vi "Average.vi"(0 "Sonar name":string) -> (7 "Sum":dbl[](array[numeric]), 8 "Average":dbl)   [LabVIEW 2017]
uses:
  <vilib>/Rock Robotics/WPI/Ultrasonic/WPI_SonarMB1010AnalogRefNum Registry Get.vi
panel:
  # "Takes 10 numbers"
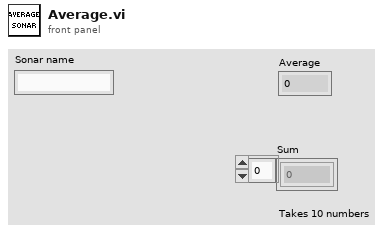
[diagram p1: front panel]
types:
  T1 = typedef "WPI_SonarMB1010AnalogDeviceRef.ctl" = cluster{"AIDeviceRef":T2, "Scaling factor (V/in)":dbl, "Average Bits":u8}
  T2 = typedef "WPI_AnalogChannelDevRef.ctl" = cluster{"DevStatus":errorcluster, "Analog Channel":T3}
  T3 = typedef "FPGA_AIChannel.ctl" = enum8{"AI 0", "AI 1", "AI 2", "AI 3", "AI MXP 0", "AI MXP 1", "AI MXP 2", "AI MXP 3", "Invalid"}
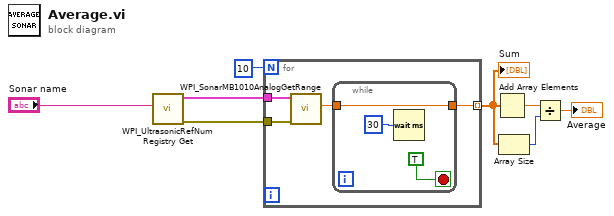
[diagram p0: block diagram]
diagram:
  n1 = call-poly <vilib>:"WPI_UltrasonicRefNum Registry Get.vi"("refnum name"="Sonar name") -> ("error out"=w3:errorcluster, "SonarMB1010AnalogDevRef"=w2:T1)  [unwired: 9 in]
  n2 = for {
    N: 10 -> [_]
    tunnel: [w12] -> w7 mode=indexing
    tunnel: w3 -> [w11]
    tunnel: w2 -> [w10]
    n3 = call "WPI_SonarMB1010AnalogGetRange.vi"("error in"=w11, "SonarMB1010AnalogDevRef"=w10) -> ("Distance"=w9:dbl)  [unwired: 7 in, 2 out]
    n4 = while {
      tunnel: w9 -> [w15]
      tunnel: [w15] -> w12
      stop <- TRUE stop-if-true
      n5 = Wait (ms)(milliseconds to wait=u32 30) -> ()  [unwired: 1 out]
    }
  }
  "Sum" <- w7
  n6 = Add Array Elements(numeric array=w7) -> (sum=w6:dbl)
  n7 = Array Size(array=w7) -> (size(s)=w5:i32)
  n8 = Divide(x=w6, y=w5) -> (x/y=→"Average":dbl)
